vi "Teleop.vi"(10 "Match Info":T2={"Autonomous Elapsed Seconds"=0.0, "TeleOp Elapsed Seconds"=0.0, "Disabled Elapsed Seconds"=0.0, "Visited Autonomous"=FALSE, "Visited TeleOp"=FALSE, "Visited Disabled"=FALSE, "Autonomous Settings"={"Autonomous Style"=enum."Independent", "VI Refnum"=refnum}}, 11 "Call Context":T3) -> ()   [LabVIEW 2014]
doc: "This VI is called for each TeleOp packet received from the DS where the robot is not disabled. It is often used to read from the joysticks and update I/O or to update setpoints for timed control loops. It should complete and return within 20 milliseconds or it may miss DS packets."
uses:
  <vilib>/Rock Robotics/WPI/DriverStation/WPI_DriverStationDerivedRobotMode.ctl
  <vilib>/Rock Robotics/WPI/DriverStation/WPI_DriverStationMatch Info.ctl
  <vilib>/Rock Robotics/WPI/Joystick/WPI_JoystickGetSetRefNum.vi
  <vilib>/Rock Robotics/WPI/RobotDrive/WPI_RobotDriveGetSetRefNum.vi
  GyroGlobal.vi
  <vilib>/addons/control/pid/pid.llb/PID (DBL).vi
  <vilib>/Rock Robotics/Network Tables/SD Write Numeric Array.vi
  <vilib>/addons/control/pid/NI_PID_pid.lvlib
panel:
  in  "Output":dbl
  out "Right":dbl(graph)
  out "Left":dbl(graph)
  in  "Strafe Lim":dbl=0.4
  in  "Speed Lim":dbl=0.7
  in  "band":dbl=0.08 format="%#_13g"
  out "Motor Outputs":cluster{"Gyro Angle":dbl, "Gyro Angle":dbl}(graph)
  out "PID Out":dbl(graph)
  out "Set and Angle":cluster{"Gyro Angle":dbl, "Gyro Angle":dbl}(graph)
  in  "PID gains":T1={"proportional gain (Kc)"=0.08, "integral time (Ti, min)"=0.0, "derivative time (Td, min)"=0.0} {"derivative time (Td, min)" format="%.3f"; "integral time (Ti, min)" format="%.3f"; "proportional gain (Kc)" format="%.3f"}
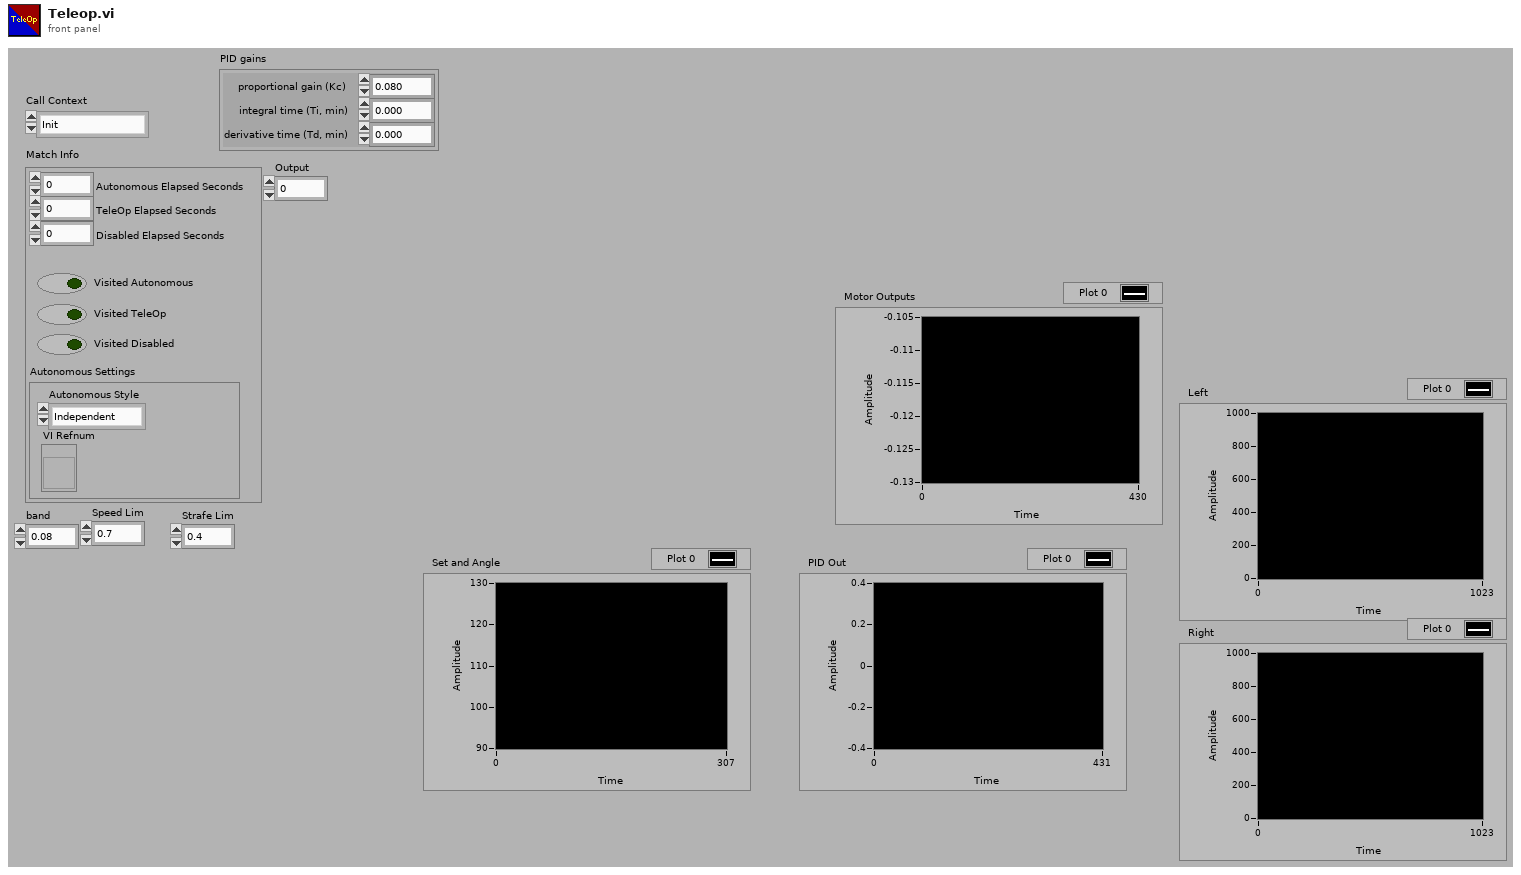
[diagram p1: front panel]
types:
  T1 = cluster{"proportional gain (Kc)":dbl, "integral time (Ti, min)":dbl, "derivative time (Td, min)":dbl}
  T2 = typedef "WPI_DriverStationMatch Info.ctl" = cluster{"Autonomous Elapsed Seconds":dbl, "TeleOp Elapsed Seconds":dbl, "Disabled Elapsed Seconds":dbl, "Visited Autonomous":bool, "Visited TeleOp":bool, "Visited Disabled":bool, "Autonomous Settings":cluster{"Autonomous Style":enum16{"Iterative", "Independent"}, "VI Refnum":refnum<vi>}}
  T3 = typedef "WPI_DriverStationDerivedRobotMode.ctl" = enum16{"Init", "Execute", "Stop"}
  T4 = typedef "WPI_JoystickDevRef.ctl" = cluster{"Device":T5}
  T5 = typedef "WPI_JoystickDeviceEnum.ctl" = enum16{"USB 0", "USB 1", "USB 2", "USB 3", "USB 4", "USB 5"}
  T6 = typedef "WPI_MotorControlDeviceRef.ctl" = cluster{"DeviceStatus":errorcluster, "Type":T7, "PWM":cluster{"Controller":T8, "PWM Channel":T9, "DeadBand":T10}, "CAN":cluster{"Device Number":u8, "Control Mode":T11, "Semaphore":T12, "Max Vout":dbl, "TalonSRX Control Mode":T13}, "Invert":bool, "TransformRef":T14, "InvTransformRef":T14}
  T7 = typedef "WPI_MotorControlType.ctl" = enum16{"PWM", "CAN", "CANTalonSRX"}
  T8 = typedef "FPGA_TypedefDigitalModule.ctl" = enum16{"Controller 1"}
  T9 = typedef "FPGA_DIOPWMChannel.ctl" = enum8{"PWM 0", "PWM 1", "PWM 2", "PWM 3", "PWM 4", "PWM 5", "PWM 6", "PWM 7", "PWM 8", "PWM 9", "PWM MXP 0", "PWM MXP 1", "PWM MXP 2", "PWM MXP 3", "PWM MXP 4", "PWM MXP 5", "PWM MXP 6", "PWM MXP 7", "PWM MXP 8", "PWM MXP 9", "Invalid"}
  T10 = typedef "WPI_PWMDeadband.ctl" = cluster{"Name":string, "maxPositivePwm":i32, "minPositivePwm":i32, "centerPwm":i32, "maxNegativePwm":i32, "minNegativePwm":i32, "angularRange":u16}
  T11 = typedef "WPI_CANJaguar_ControlMode.ctl" = enum8{"Percent VBus", "Current", "Speed", "Position", "Voltage"}
  T12 = typedef "Semaphore RefNum" = refnum<k1>
  T13 = typedef "WPI_CANTalonSRX_APIControlMode.ctl" = enum8{"Percent VBus", "Speed", "Position", "Slave", "Unchanged / Invalid"}
  T14 = typedef "WPI_PWMTransform_ConPane.ctl" = refnum<vi>
  T15 = typedef "WPI_CANTalonSRX_GlobalStatus.ctl" = cluster{"Applied Throttle":dbl, "Module Enabled":bool, "CAN Error":errorcluster, "Closed Loop Error":dbl, "Forward Limit Switch Closed":bool, "Reverse Limit Switch Closed":bool, "Sensor Position":dbl, "Sensor Velocity":dbl, "Current":dbl, "Sticky Fault - Over Temp":bool, "Sticky Fault - Under Voltage":bool, "Sticky Fault - Forward Limit":bool, "Sticky Fault - Reverse Limit":bool, "Sticky Fault - Forward Soft Limit":bool, "Sticky Fault - Reverse Soft Limit":bool, "Brake is Enabled":bool, "Encoder Position":dbl, "Encoder Velocity":dbl, "Encoder Index Count":dbl, "Encoder A Pin State":bool, "Encoder B Pin State":bool, "Encoder Index Pin State":bool, "Analog In":dbl, "Analog In Velocity":dbl, "Temperature (C)":dbl, "Battery Voltage":dbl}
  T16 = typedef "WPI_RobotDriveDevRef.ctl" = cluster{"DevStatus":errorcluster, "Motors[]":T6[], "Square Inputs":bool, "Max Output":dbl}
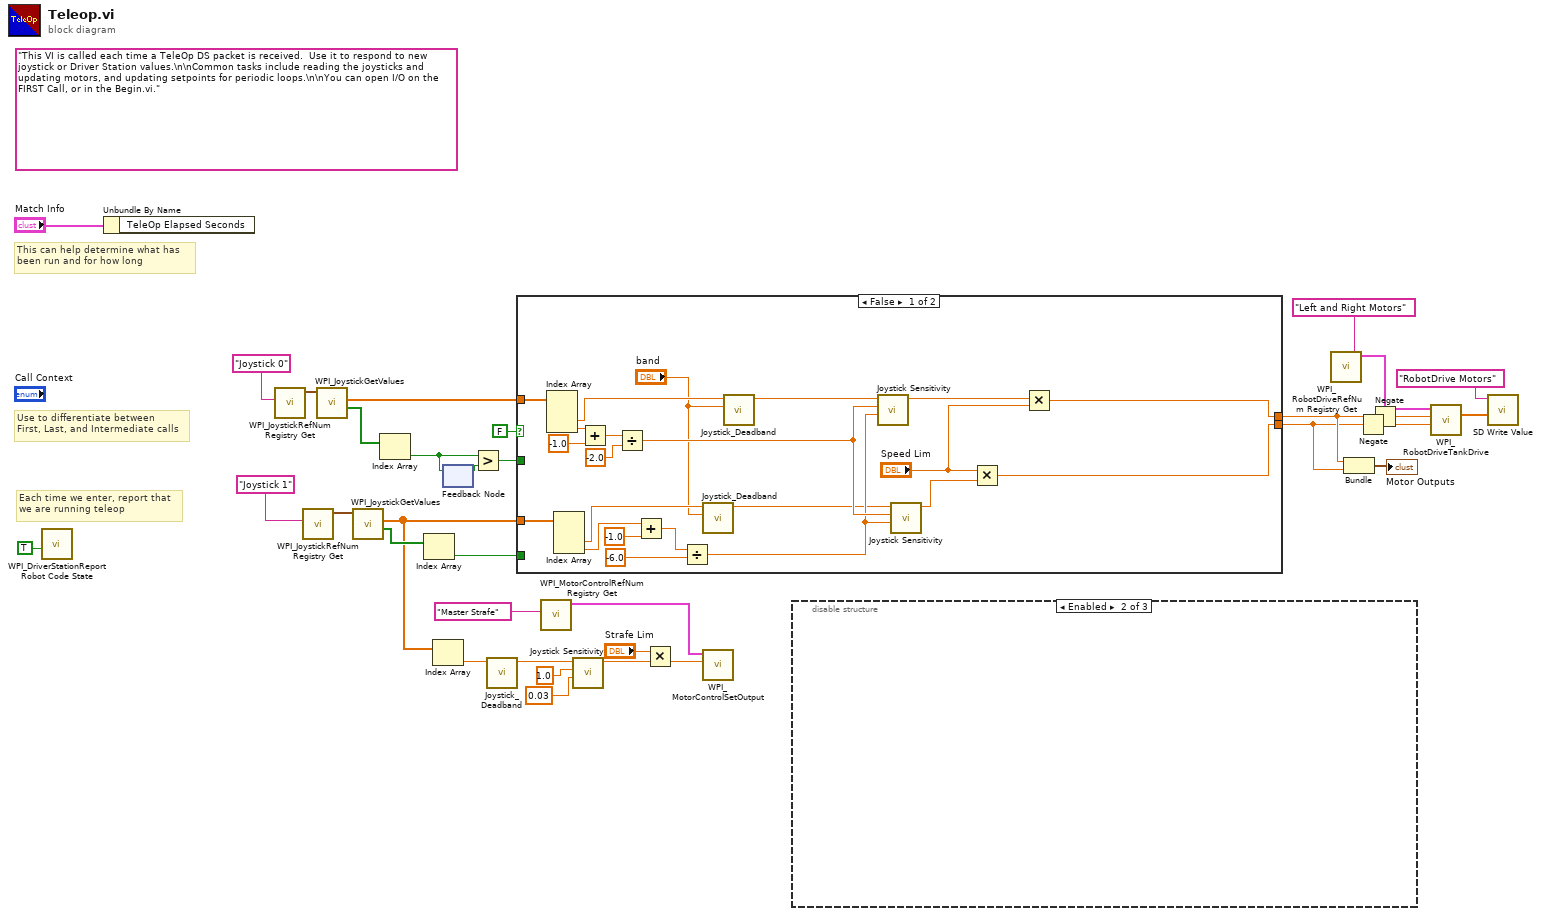
[diagram p0: block diagram]
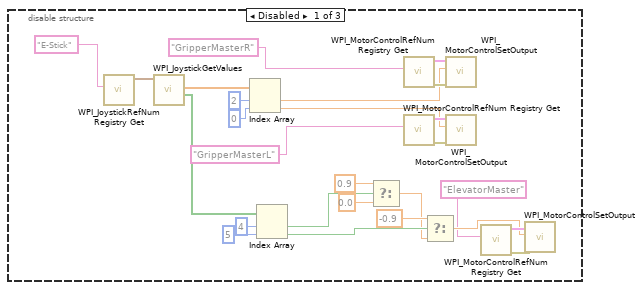
[diagram p2: hidden frame]
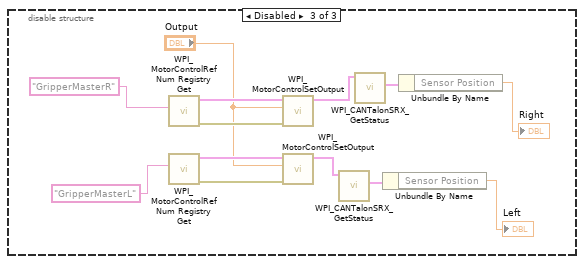
[diagram p3: hidden frame]
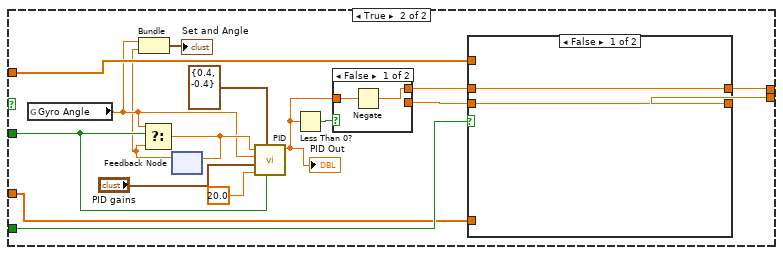
[diagram p4: hidden frame]
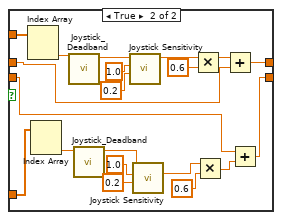
[diagram p5: hidden frame]
diagram:
  (unwired) "This VI is called each time a TeleOp DS packet is received.  Use it to respond to new joystick or Driver Station values.\n\nCommon tasks include reading the joysticks and updating motors, and updating setpoints for periodic loops.\n\nYou can open I/O on the FIRST Call, or in the Begin.vi."
  # "Each time we enter, report that\nwe are running teleop"
  # "Use to differentiate between\nFirst, Last, and Intermediate calls"
  # "This can help determine what has\nbeen run and for how long"
  n1 = call <vilib>:"WPI_DriverStationReport Robot Code State.vi"("TeleOp"=TRUE ("Autonomous")) -> ()  [unwired: 10 in, 1 out]
  n2 = Unbundle By Name("Match Info") -> ()  [unwired: 1 out]
  n3 = call <vilib>:"WPI_JoystickRefNum Registry Get.vi"("refnum name"="Joystick 0") -> ("JoystickDevRef"=w30:T4)  [unwired: 1 in, 9 out]
  n4 = call <vilib>:"WPI_JoystickRefNum Registry Get.vi"("refnum name"="Joystick 1") -> ("JoystickDevRef"=w24:T4)  [unwired: 1 in, 9 out]
  n5 = call <vilib>:"WPI_JoystickGetValues.vi"("JoystickDevRef"=w30) -> ("Buttons"=w28:bool[], "Axes"=w29:dbl[])  [unwired: 6 in, 3 out]
  n6 = call <vilib>:"WPI_JoystickGetValues.vi"("JoystickDevRef"=w24) -> ("Buttons"=w18:bool[], "Axes"=w9:dbl[])  [unwired: 6 in, 3 out]
  n7 = Index Array(array=w28) -> (element=w26:bool)  [unwired: 1 in]
  n8 = Index Array(array=w18) -> (element=w17:bool)  [unwired: 1 in]
  n9 = Index Array(array=w9) -> (element=w7:dbl)  [unwired: 1 in]
  n10 = feedback #1() -> (w27:bool)  [unwired: 1 in]
  n11 = feedback-in #1(w26) -> ()
  n12 = Greater?(x=w26, y=w27) -> (0:w25:bool)
  n13 = call "Joystick_Deadband.vi"("in"=w7) -> ("out"=w10:dbl)  [unwired: 10 in]
  n14 = case shown="False" FALSE {
    tunnel: w29 -> [w55 w61]
    tunnel: w25 -> [_ w69]
    tunnel: w9 -> [w54 w60]
    tunnel: [w35 w64] -> w15
    tunnel: [w37 w63] -> w14
    tunnel: w17 -> [_ w62]
    frame False {
      n15 = Index Array(array=w55) -> (element #2=w42:dbl, element #3=w52:dbl)  [unwired: 3 in, 1 out]
      n16 = Index Array(array=w54) -> (element #2=w41:dbl, element #3=w46:dbl)  [unwired: 3 in, 1 out]
      n17 = Add(x=w52, y=-1.0) -> (x+y=w51:dbl)
      n18 = Divide(x=w51, y=-2.0) -> (x/y=w49:dbl)
      n19 = Add(x=w46, y=-1.0) -> (x+y=w45:dbl)
      n20 = Divide(x=w45, y=-6.0) -> (x/y=w44:dbl)
      n21 = call "Joystick_Deadband.vi"("band"="band", "in"=w41) -> ("out"=w40:dbl)  [unwired: 9 in]
      n22 = call "Joystick_Deadband.vi"("band"="band", "in"=w42) -> ("out"=w43:dbl)  [unwired: 9 in]
      n23 = call "Joystick Sensitivity.vi"("B"=w44, "A"=w49, "X"=w43) -> ("Y"=w36:dbl)  [unwired: 8 in]
      n24 = call "Joystick Sensitivity.vi"("B"=w44, "A"=w49, "X"=w40) -> ("Y"=w38:dbl)  [unwired: 8 in]
      n25 = Multiply(x="Speed Lim", y=w38) -> (x*y=w37:dbl)
      n26 = Multiply(x=w36, y="Speed Lim") -> (x*y=w35:dbl)
    }
    frame True {
      n27 = global read "GyroGlobal.vi" "Gyro Angle"() -> (w57:dbl)
      n28 = feedback #2() -> (w56:dbl)  [unwired: 1 in]
      n29 = Bundle("Gyro Angle"=w57, "Gyro Angle"=w56) -> (→"Set and Angle":cluster{"Gyro Angle":dbl, "Gyro Angle":dbl})  [unwired: 1 in]
      n30 = Select(t=w57, s=w69, f=w56) -> (s? t:f=w68:dbl)
      n31 = feedback-in #2(w68) -> ()
      n32 = call-poly <vilib>:"PID.vi"("reinitialize? (F)"=w69, "output range"=cluster{"output high":dbl, "output low":dbl} {"output high"=0.4, "output low"=-0.4}, "dt (s)"=20.0, "PID gains"="PID gains", "process variable"=w57, "setpoint"=w68) -> ("output"=w59:dbl)  [unwired: 4 in, 1 out]
      "PID Out" <- w59
      n33 = Less Than 0?(x=w59) -> (x < 0?=w70:bool)
      n34 = case shown="False" w70 {
        tunnel: w59 -> [w96 w97]
        tunnel: [_ w97] -> w65
        tunnel: [w95 _] -> w66
        frame False {
          n35 = Negate(x=w96) -> (-x=w95:dbl)
        }
        frame True {
        }
      }
      n36 = case shown="False" w62 {
        tunnel: w66 -> [w74 w84]
        tunnel: w65 -> [w73 w85]
        tunnel: [w74 w83] -> w64
        tunnel: [w73 w82] -> w63
        tunnel: w61 -> [_ w94]
        tunnel: w60 -> [_ w93]
        frame False {
        }
        frame True {
          n37 = Index Array(array=w94) -> (element #2=w81:dbl)  [unwired: 2 in, 1 out]
          n38 = Index Array(array=w93) -> (element #2=w78:dbl)  [unwired: 2 in, 1 out]
          n39 = call "Joystick_Deadband.vi"("in"=w81) -> ("out"=w92:dbl)  [unwired: 10 in]
          n40 = call "Joystick_Deadband.vi"("in"=w78) -> ("out"=w91:dbl)  [unwired: 10 in]
          n41 = call "Joystick Sensitivity.vi"("B"=0.2, "A"=1.0, "X"=w92) -> ("Y"=w86:dbl)  [unwired: 8 in]
          n42 = call "Joystick Sensitivity.vi"("B"=0.2, "A"=1.0, "X"=w91) -> ("Y"=w77:dbl)  [unwired: 8 in]
          n43 = Multiply(x=w86, y=0.6) -> (x*y=w80:dbl)
          n44 = Multiply(x=w77, y=0.6 ("x")) -> (x*y=w76:dbl)
          n45 = Add(x=w80, y=w84) -> (x+y=w83:dbl)
          n46 = Add(x=w85, y=w76) -> (x+y=w82:dbl)
        }
      }
    }
  }
  n47 = call <vilib>:"WPI_MotorControlRefNum Registry Get.vi"("refnum name"="Master Strafe") -> ("MotorControlDevRef"=w6:T6)  [unwired: 9 in, 1 out]
  n48 = call "Joystick Sensitivity.vi"("B"=0.03, "A"=1.0, "X"=w10) -> ("Y"=w5:dbl)  [unwired: 8 in]
  n49 = Multiply(x="Strafe Lim", y=w5) -> (x*y=w2:dbl)
  n50 = call <vilib>:"WPI_MotorControlSetOutput.vi"("Output"=w2, "MotorControlDevRef"=w6) -> ()  [unwired: 7 in, 3 out]
  n51 = disable-structure shown="Enabled" {
    frame Disabled {
      n52 = call <vilib>:"WPI_JoystickRefNum Registry Get.vi"("refnum name"="E-Stick") -> ("JoystickDevRef"=w123:T4)  [unwired: 1 in, 9 out]
      n53 = call <vilib>:"WPI_JoystickGetValues.vi"("JoystickDevRef"=w123) -> ("Buttons"=w118:bool[], "Axes"=w121:dbl[])  [unwired: 6 in, 3 out]
      n54 = Index Array(array=w121, index #1=2 ("index"), index #2=0 ("index")) -> (element #1=w98:dbl, element #2=w99:dbl)
      n55 = Index Array(array=w118, index #1=4 ("index"), index #2=5 ("index")) -> (element #1=w115:bool, element #2=w112:bool)
      n56 = Select(t=0.9, s=w115, f=0.0) -> (s? t:f=w110:dbl)
      n57 = call <vilib>:"WPI_MotorControlRefNum Registry Get.vi"("refnum name"="GripperMasterR") -> ("error out"=w102:errorcluster, "MotorControlDevRef"=w103:T6)  [unwired: 9 in]
      n58 = call <vilib>:"WPI_MotorControlRefNum Registry Get.vi"("refnum name"="GripperMasterL") -> ("error out"=w100:errorcluster, "MotorControlDevRef"=w101:T6)  [unwired: 9 in]
      n59 = Select(t=-0.9, s=w112, f=w110) -> (s? t:f=w107:dbl)
      n60 = call <vilib>:"WPI_MotorControlSetOutput.vi"("error in (no error)"=w102, "Output"=w98, "MotorControlDevRef"=w103) -> ()  [unwired: 6 in, 3 out]
      n61 = call <vilib>:"WPI_MotorControlSetOutput.vi"("error in (no error)"=w100, "Output"=w99, "MotorControlDevRef"=w101) -> ()  [unwired: 6 in, 3 out]
      n62 = call <vilib>:"WPI_MotorControlRefNum Registry Get.vi"("refnum name"="ElevatorMaster") -> ("error out"=w109:errorcluster, "MotorControlDevRef"=w108:T6)  [unwired: 9 in]
      n63 = call <vilib>:"WPI_MotorControlSetOutput.vi"("error in (no error)"=w109, "Output"=w107, "MotorControlDevRef"=w108) -> ()  [unwired: 6 in, 3 out]
    }
    frame Enabled {
    }
    frame Disabled {
      n64 = call <vilib>:"WPI_MotorControlRefNum Registry Get.vi"("refnum name"="GripperMasterR") -> ("error out"=w131:errorcluster, "MotorControlDevRef"=w132:T6)  [unwired: 9 in]
      n65 = call <vilib>:"WPI_MotorControlRefNum Registry Get.vi"("refnum name"="GripperMasterL") -> ("error out"=w129:errorcluster, "MotorControlDevRef"=w130:T6)  [unwired: 9 in]
      n66 = call <vilib>:"WPI_MotorControlSetOutput.vi"("error in (no error)"=w131, "Output"="Output", "MotorControlDevRef"=w132) -> ("MotorControlDevRef"=w126:T6)  [unwired: 6 in, 2 out]
      n67 = call <vilib>:"WPI_MotorControlSetOutput.vi"("error in (no error)"=w129, "Output"="Output", "MotorControlDevRef"=w130) -> ("MotorControlDevRef"=w125:T6)  [unwired: 6 in, 2 out]
      n68 = call <vilib>:"WPI_CANTalonSRX_GetStatus.vi"("CAN Talon SRX Ref"=w125) -> ("Talon SRX Status"=w136:T15)  [unwired: 8 in, 2 out]
      n69 = call <vilib>:"WPI_CANTalonSRX_GetStatus.vi"("CAN Talon SRX Ref"=w126) -> ("Talon SRX Status"=w127:T15)  [unwired: 8 in, 2 out]
      n70 = Unbundle By Name(w136) -> ("Sensor Position"=→"Left":dbl)
      n71 = Unbundle By Name(w127) -> ("Sensor Position"=→"Right":dbl)
    }
  }
  n72 = call <vilib>:"WPI_RobotDriveRefNum Registry Get.vi"("refnum name"="Left and Right Motors") -> ("RobotDriveDevRef"=w20:T16)  [unwired: 1 in, 9 out]
  n73 = Bundle(w15, "output"=w14) -> (→"Motor Outputs":cluster{dbl, "output":dbl})  [unwired: 1 in]
  n74 = Negate(x=w14) -> (-x=w4:dbl)
  n75 = Negate(x=w15) -> (-x=w3:dbl)
  n76 = call <vilib>:"WPI_RobotDriveTankDrive.vi"("Right axis value"=w4, "Left axis value"=w3, "RobotDriveDevRef"=w20) -> ("Motor Values"=w22:dbl[])  [unwired: 6 in, 2 out]
  n77 = call-poly <vilib>:"SD Write Value.vi"("Numeric Array"=w22, "Name"="RobotDrive Motors") -> ()  [unwired: 8 in, 2 out]
